vi "Get Resource Type.vi"(4 "SPI CS in":refnum<class "SPI CS.lvclass">) -> (7 "Resource Type":string)   [LabVIEW 2024, in "CTI.lvlib" / "SPI CS.lvclass"]
uses:
  SPI CS.lvclass
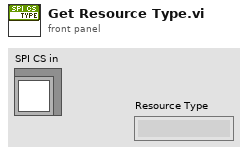
[diagram p1: front panel]
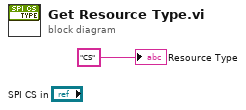
[diagram p0: block diagram]
diagram:
  "Resource Type" <- "CS" ("Resource Type")
